vi "TLB Native Dynamic Events ver 0.07.vi"() -> ()   [LabVIEW 2018]
uses:
  Labview Training Phase 2/Enum Controls/States for Action Engine.ctl
  Type def/TLB event states.ctl
  Type def/TLB MHL States.ctl
  <vilib>/Studica/Studica Toolkit/Background/I2C Channel.ctl
  <vilib>/Studica/Studica Toolkit/NavX/NavX.lvlib
  <vilib>/myRIO/Common/Instrument Driver Framework/myRIO v1.0/AI/typedefs/AI Channels Enum.ctl
  <vilib>/myRIO/Common/Instrument Driver Framework/myRIO v1.0/AI/typedefs/AI Channels List.ctl
  Type def/Type def.ctl
  Type def/Motor Control Cluster.ctl
  <vilib>/Studica/Studica Blackhawk/Blackhawk.lvlib
  <vilib>/userdefined/High Color/IMAQdx.ctl
  Underlying VI's/Webcam FGV Low level ver/State control.ctl
  <vilib>/Studica/Studica Toolkit/Background/Mxp Selection.ctl
  <vilib>/ptbypt/NI_PtbyPt.lvlib
  <vilib>/Studica/Studica Toolkit/Background/DIO Channel.ctl
  <vilib>/addons/control/pid/NI_PID_pid.lvlib
  <vilib>/addons/control/pid/pid.llb/PID (DBL).vi
panel:
  in  "STOP":bool
  out "DIO 0":bool
  out "DIO 1":bool
  out "Limit Switch Array":bool[](array[boolean])
  out "Speed and distance cluster":T1
  out "error out":errorcluster
  out "Blackhawk loop":i32
  out "NavX Loop":i32
  out "Sensor Loop":i32
  out "User event loop":i32
  out "Event handling loop":i32
  out "Main Loop":i32
  out "Status loop":i32
  out "L/R average":fxp<+,64,64>
  out "Right Ultrasonic":fxp<+,64,16>
  out "Left Ultrasonic":fxp<+,64,16>
  out "Object detection count":T2
  out "Camera error":errorcluster
  out "Right IR Sensor":dbl
  out "Left IR Sensor":dbl
  in  "Servo Angle":u8(slide) scale=0.0..180.0
  in  "On/Off":bool
  out "Blackhawk error":errorcluster
  out "Image Out":T3(plugin-control)
  out "element":T4
  out "Action Queue Items":i32
  out "State Logic Queue Items":i32
  out "Action Queues items":string[](array[string])=["Hardware reset", "Software reset", ""]
  out "State logic":T5=enum."Task 2"
  out "Action State":string
  in  "Tasks Selector":string(combo)="Wall following"
  out "Yaw":dbl
  out "NavX Info Out":T7
  out "LinearAcceleration":T8
  out "Displacement":T9
  out "YRPHfH":T10
  out "Object detected":bool
  in  "NavX Zero Yaw":bool
  # "Camera Status Loop"
  # "TLB FRAMEWORK STATUS"
  # "Test Programme written by Calvin Loke    Dated: 28 Aug 2019\nTest Programme revised by Dr Alex See   Dated 30 Aug 2019\n\nProgramme version:   TLB Native Dynamic Events ver 0.04b.vi"
  # "Sequence of Actions"
  # "Continuous (Repeated)"
  # "Motor Control Loop"
  # "Sensor data"
  # "Blackhawk status"
  # "System Health Status Update"
  # "NAVX Control Loop"
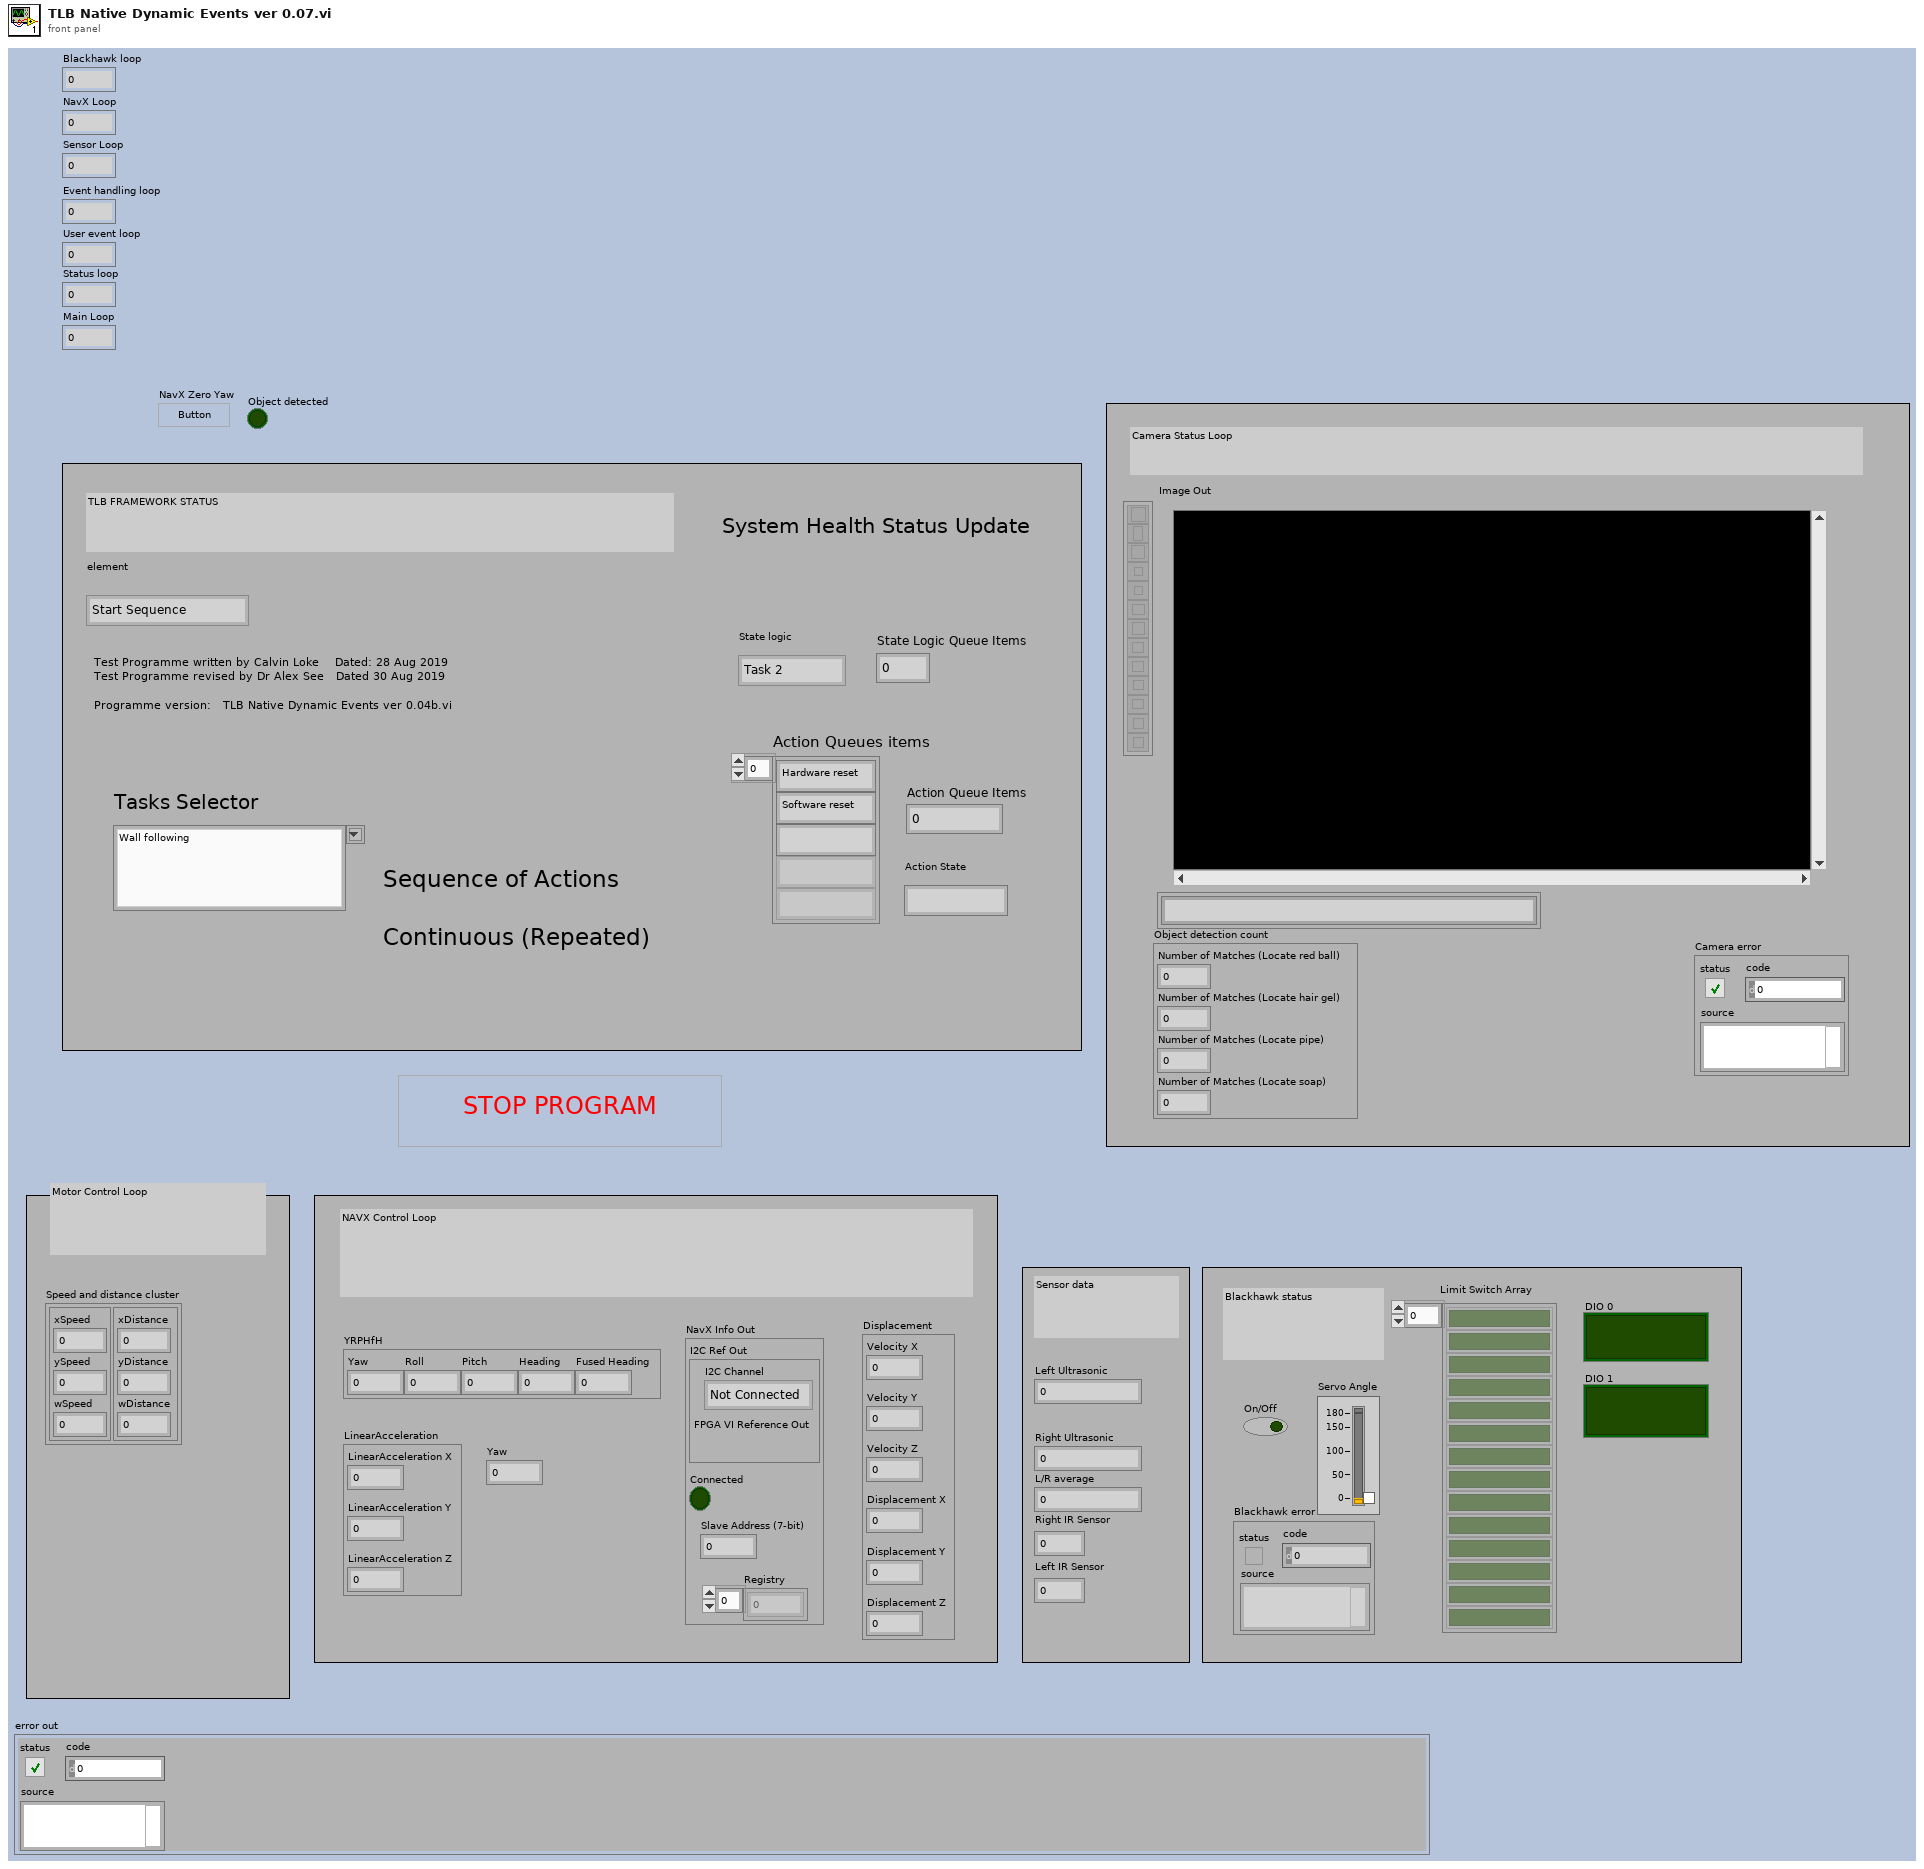
[diagram p1: front panel]
types:
  T1 = cluster{cluster{"xSpeed":dbl, "ySpeed":dbl, "wSpeed":dbl}, cluster{"xDistance":dbl, "yDistance":dbl, "wDistance":dbl}}
  T2 = cluster{"Number of Matches (Locate red ball)":i32, "Number of Matches (Locate hair gel)":i32, "Number of Matches (Locate pipe)":i32, "Number of Matches (Locate soap)":i32}
  T3 = typedef "IMAQ Image.ctl" = refnum<image>
  T4 = typedef "TLB event states.ctl" = enum16{"Start Sequence", "Exit", "Start Task 1", "Start Task 2", "Start Task 3", "Start Task 4", "Camera vision", "Wall follow mode", "Idle", "Start Drive Straight"}
  T5 = typedef "TLB MHL States.ctl" = enum16{"None", "Startup", "Idle", "Processing", "Shutdown", "Reset", "Task 1", "Task 2", "Task 3", "Task 4", "Task 4a", "Task 4b", "Task 4c", "Task 4d", "Task 4e", "Task 4f", "Task 4g", "Task 4h", "Acquire image", "Wall follow mode", "Autodrive", "Autodrive a"}
  T6 = typedef "I2C Channel.ctl" = enum16{"Not Connected", "A", "B"}
  T7 = cluster{"I2C Ref Out":cluster{"I2C Channel":T6, "FPGA VI Reference Out":refnum<k20>}, "Connected":bool, "Slave Address (7-bit)":u8, "Registry":u8[]}
  T8 = cluster{"LinearAcceleration X":dbl, "LinearAcceleration Y":dbl, "LinearAcceleration Z":dbl}
  T9 = cluster{"Velocity X":dbl, "Velocity Y":dbl, "Velocity Z":dbl, "Displacement X":dbl, "Displacement Y":dbl, "Displacement Z":dbl}
  T10 = cluster{"Yaw":dbl, "Roll":dbl, "Pitch":dbl, "Heading":dbl, "Fused Heading":dbl}
  T11 = typedef "States for Action Engine.ctl" = enum16{"Initialize", "Write", "Read"}
  T12 = typedef "DIO Channel.ctl" = enum16{"Not Connected", "A/DIO1", "A/DIO2", "A/DIO3", "A/DIO4", "A/DIO5", "A/DIO6", "A/DIO7", "A/DIO13", "B/DIO1", "B/DIO2", "B/DIO3", "B/DIO4", "B/DIO5", "B/DIO6", "B/DIO7", "B/DIO13", "C/DIO0", "C/DIO1", "C/DIO2", "C/DIO3", "C/DIO4", "C/DIO5", "C/DIO6", "C/DIO7"}
  T13 = typedef "Motor Control Cluster.ctl" = cluster{"Vx":dbl, "Vy":dbl, "Vw":dbl}
  T14 = typedef "Type def.ctl" = cluster{"Front Ultrasonic Obstruct":bool, "Left Ultrasonic Obstruct":bool, "Right Ultrasonic Obstruct ":bool}
  T15 = typedef "Mxp Selection.ctl" = enum16{"MXP A", "MXP B"}
  T16 = cluster{"proportional gain (Kc)":dbl, "integral time (Ti, min)":dbl, "derivative time (Td, min)":dbl}
  T17 = typedef "State control.ctl" = enum16{"Initialise", "Start camera", "Continuous Acquisition ", "Stop camera", "Dispose all"}
  T18 = typedef "IMAQdx.ctl" = refnum<k21>
  T19 = cluster{"xTargetSpeed":dbl, "yTargetSpeed":dbl, "wTargetSpeed":dbl}
  T20 = cluster{"DIO Channel":T12, "FPGA VI Reference Out":refnum<k20>}
  T21 = cluster{"xDistance":dbl, "yDistance":dbl, "wDistance":dbl}
  T22 = typedef "AI Channels List.ctl" = T23[]
  T23 = typedef "AI Channels Enum.ctl" = enum16{"Not Connected", "AudioIn/Left", "AudioIn/Right", "C/AI0", "C/AI1", "A/AI0", "A/AI1", "A/AI2", "A/AI3", "A/AI4", "A/AI5", "A/AI6", "A/AI7", "B/AI0", "B/AI1", "B/AI2", "B/AI3", "B/AI4", "B/AI5", "B/AI6", "B/AI7", "AI/AI0", "AI/AI1", "AI/AI2", "AI/AI3", "A/AI0 (DIFF)", "A/AI1 (DIFF)", "A/AI2 (DIFF)", "A/AI3 (DIFF)", "B/AI0 (DIFF)", "B/AI1 (DIFF)", "B/AI2 (DIFF)", "B/AI3 (DIFF)"}
  T24 = cluster{"I2C Channel":T6, "FPGA VI Reference Out":refnum<k20>}
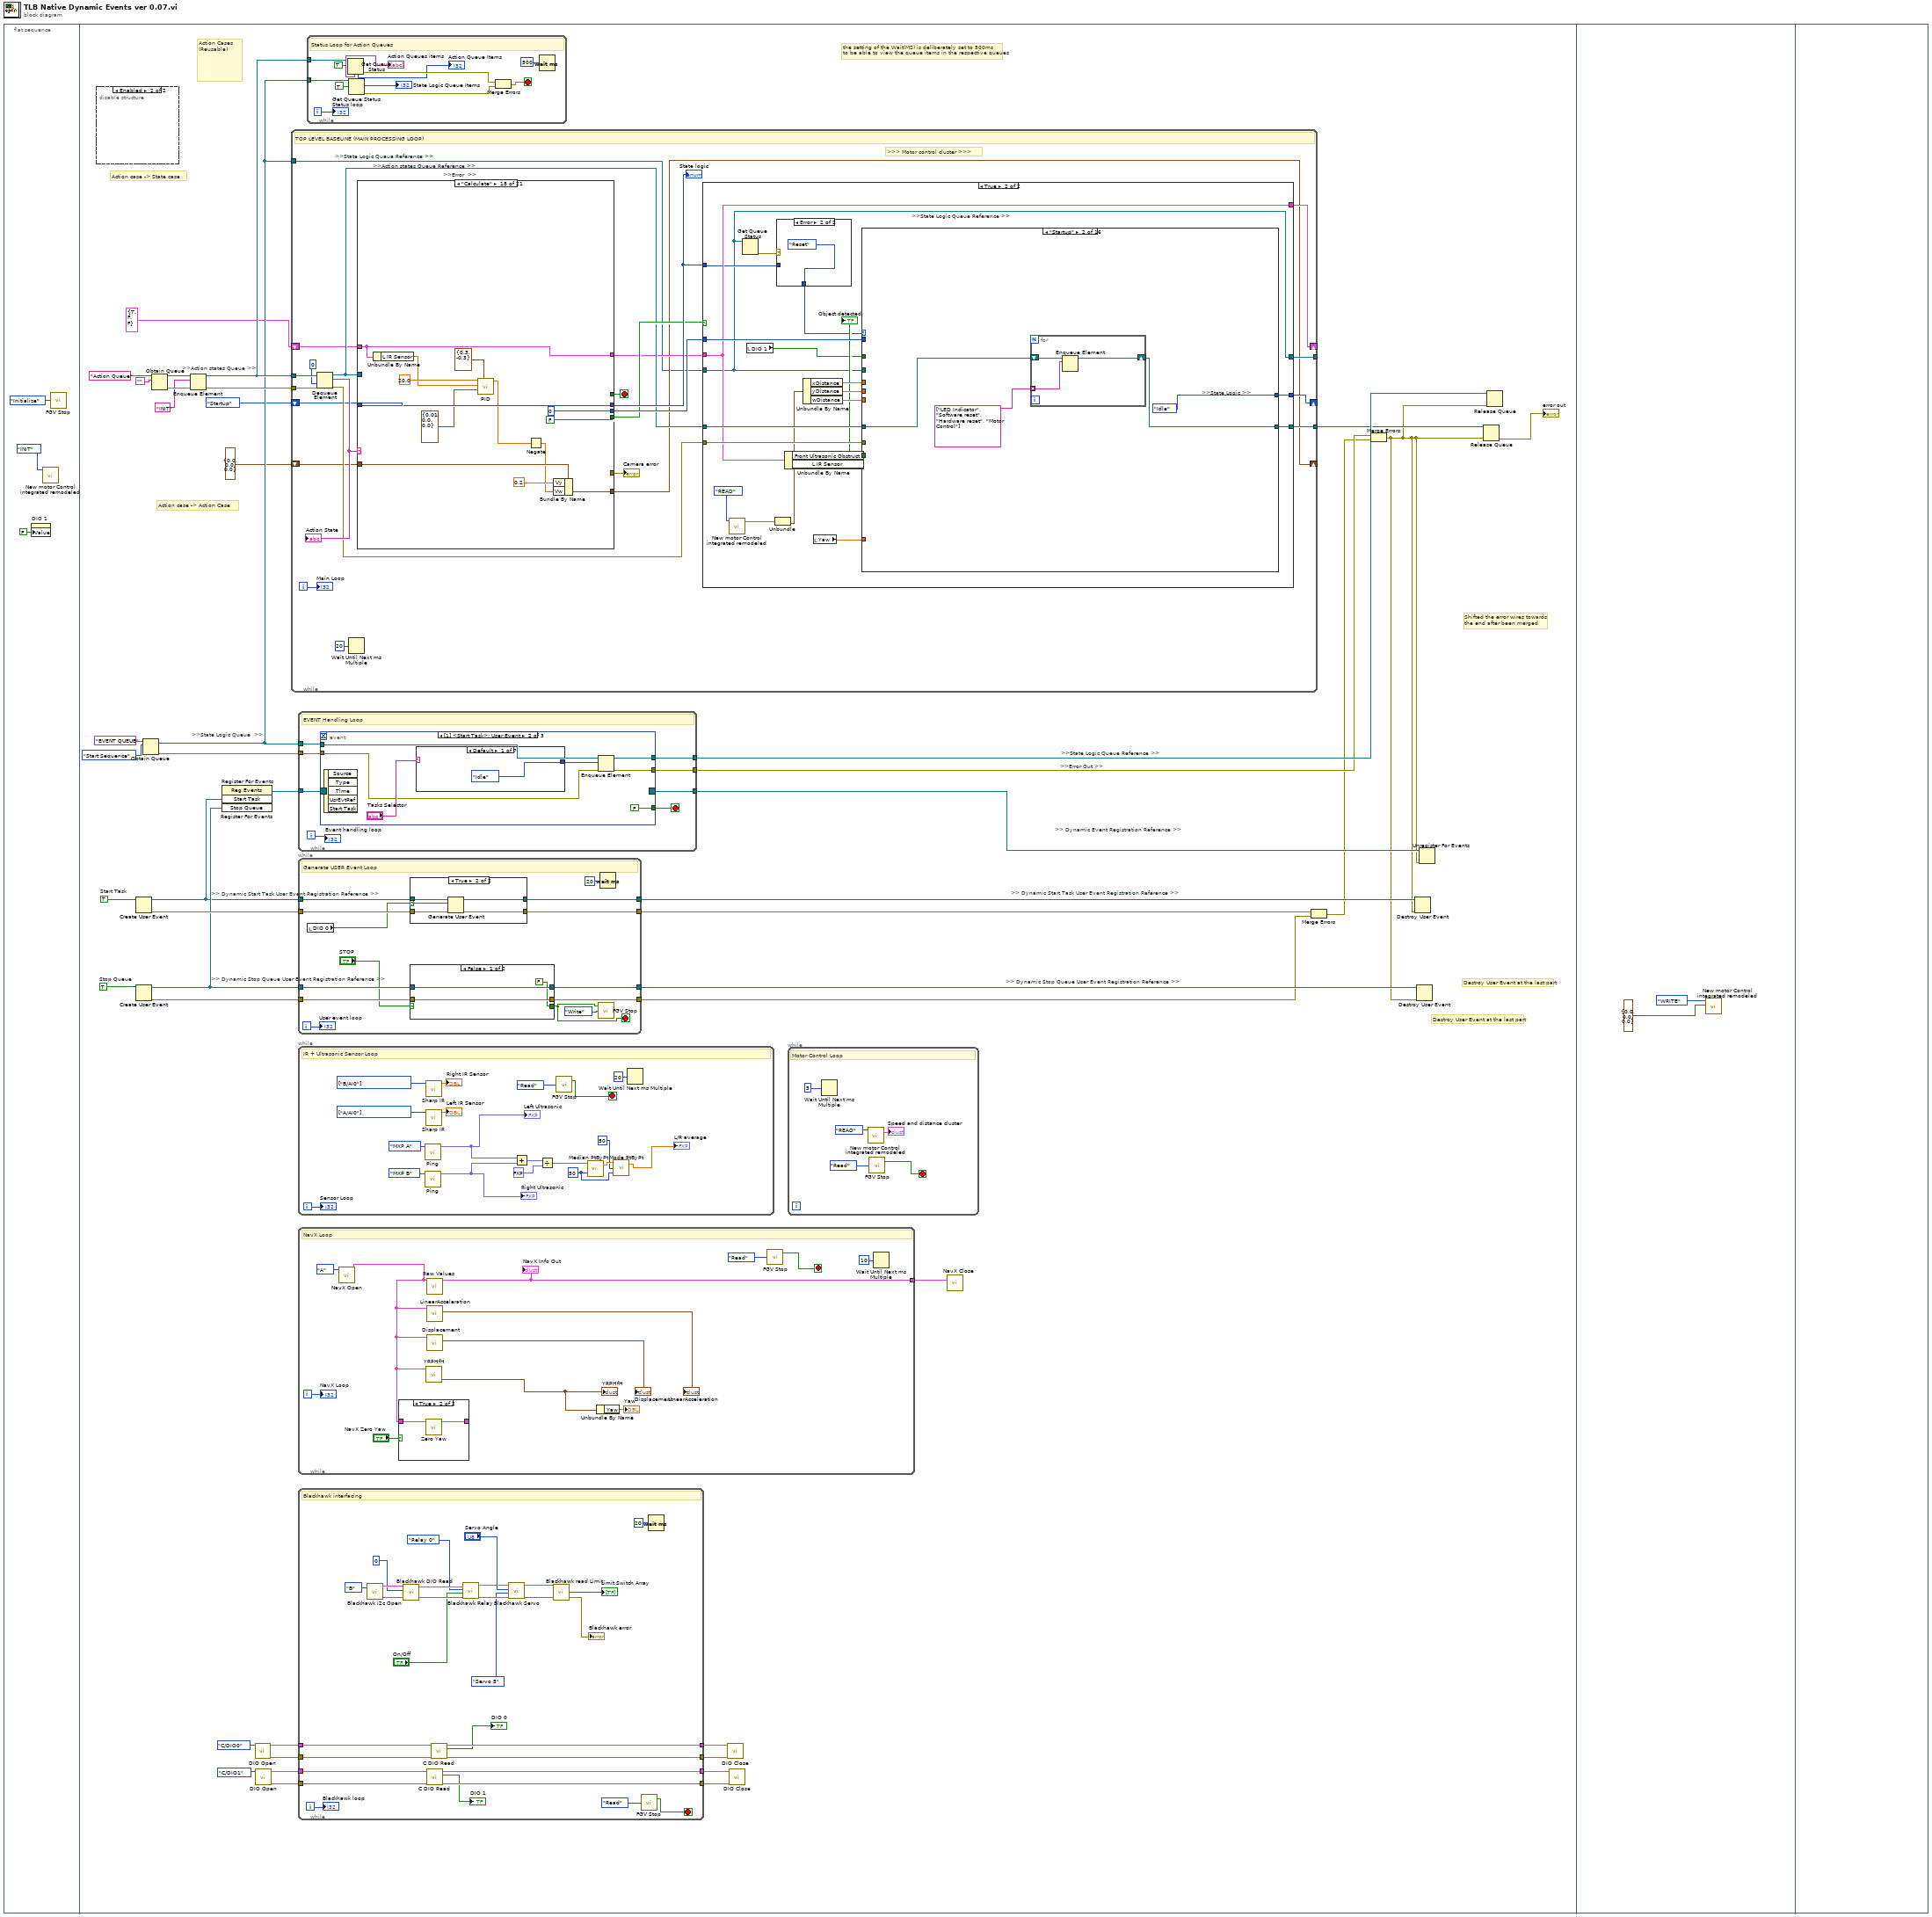
[diagram p0: block diagram]
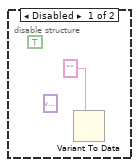
[diagram p3: hidden frame]
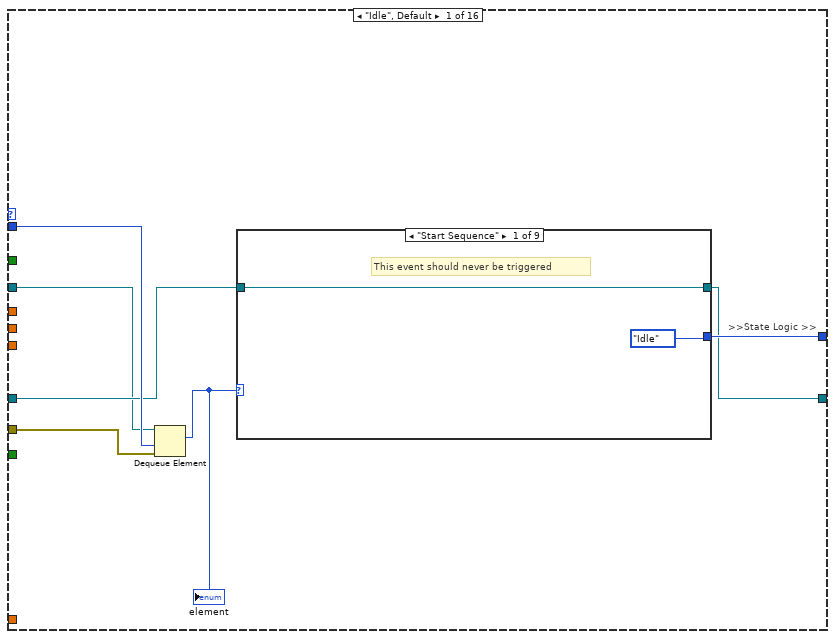
[diagram p6: hidden frame]
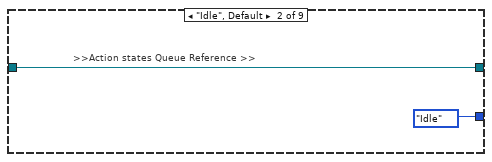
[diagram p7: hidden frame]
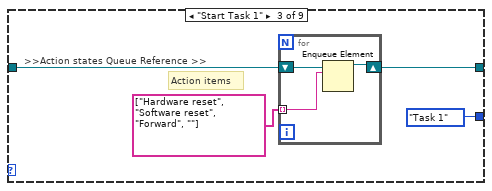
[diagram p8: hidden frame]
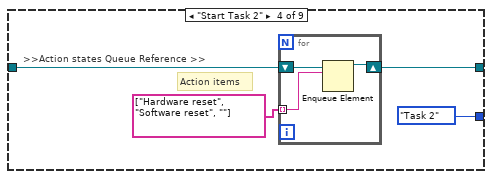
[diagram p9: hidden frame]
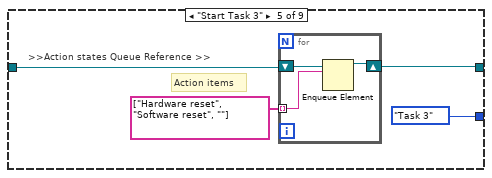
[diagram p10: hidden frame]
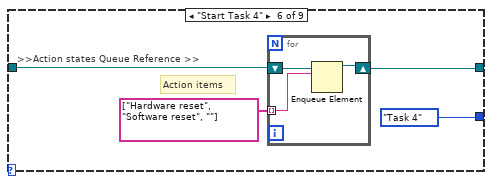
[diagram p11: hidden frame]
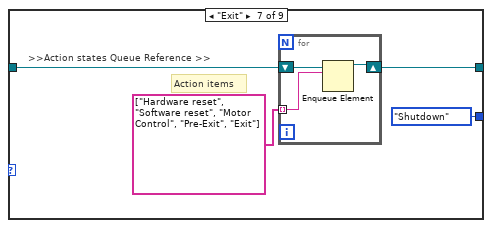
[diagram p12: hidden frame]
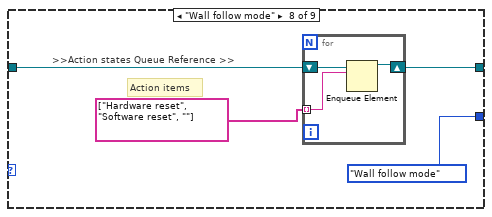
[diagram p13: hidden frame]
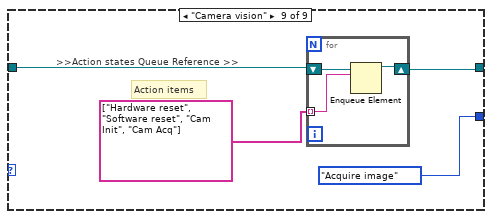
[diagram p14: hidden frame]
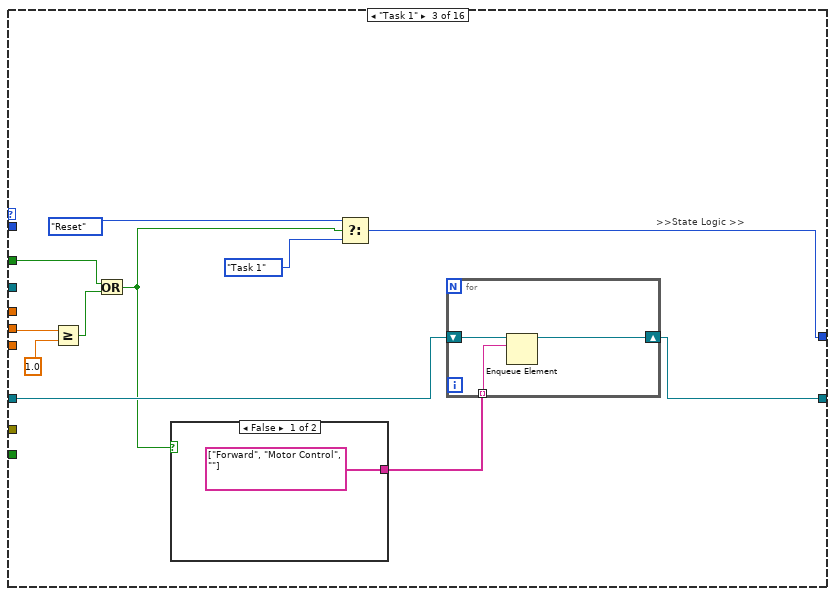
[diagram p15: hidden frame]
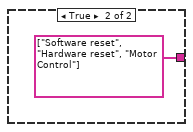
[diagram p16: hidden frame]
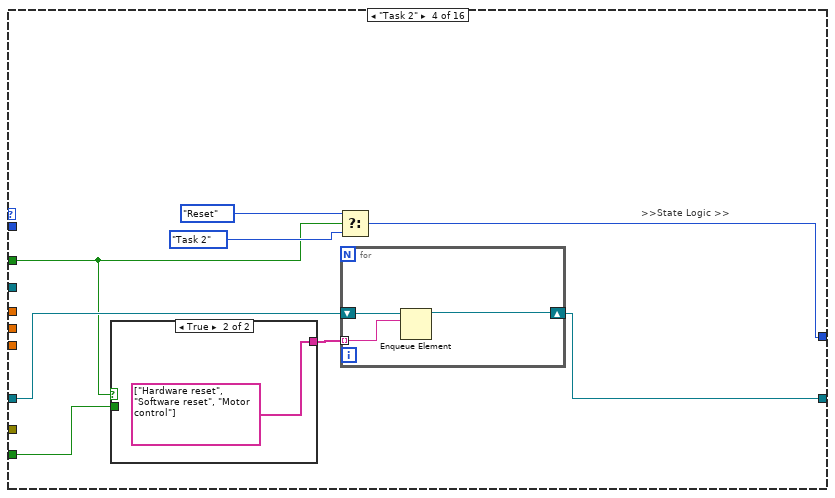
[diagram p17: hidden frame]
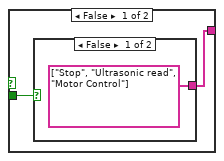
[diagram p18: hidden frame]
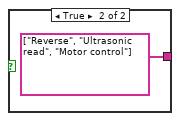
[diagram p19: hidden frame]
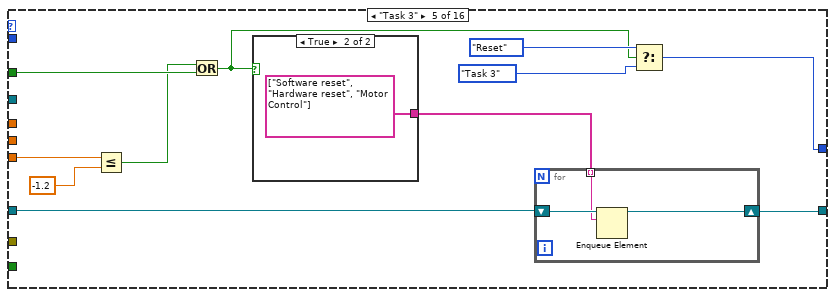
[diagram p20: hidden frame]
diagram:
  n1 = flat-sequence {
    frame #0 {
      n2 = property on="DIO 1" class="Bool (strict)"("Value"=FALSE ("DIO 1")) -> ()  [unwired: 2 in, 2 out]
      n3 = call "New motor Control integrated remodeled.vi"("States"=enum16{"RESET ENCODER", "WRITE", "READ", "INIT"}."INIT") -> ()  [unwired: 4 in, 2 out]
      n4 = call "FGV Stop.vi"("Init/Read/Write State"=States_for_Action_Engine."Initialize") -> ()  [unwired: 2 in, 2 out]
    }
    frame #1 {
      w46 = TRUE  # Stop Queue
      w45 = TRUE  # Start Task
      # "Action case -> Action Case"
      # "Action case -> State case"
      # "the setting of the Wait(MS) is deliberately set to 500ms\nto be able to view the queue items in the respective queues"
      # "Action Cases\n(Reusable)"
      # ">>Error Out >>"
      # ">> Dynamic Stop Queue User Event Registration Reference >>"
      # ">> Dynamic Start Task User Event Registration Reference >>"
      # ">> Dynamic Stop Queue User Event Registration Reference >>"
      # ">> Dynamic Start Task User Event Registration Reference >>"
      # ">> Dynamic Event Registration Reference >>"
      # ">>Action states Queue >>"
      # ">>State Logic Queue  >>"
      # ">>State Logic Queue Reference >>"
      # "Destroy User Event at the last part"
      # "Destroy User Event at the last part"
      # "Shifted the error wires towards\nthe end after been merged"
      n5 = disable-structure shown="Enabled" {
        frame Disabled {
          (unwired) variant
          (unwired) TRUE
          n6 = Variant To Data(type="") -> ()  [unwired: 2 in, 2 out]
        }
        frame Enabled {
        }
      }
      n7 = Create User Event(user event datatype=w45) -> (user event=w37:refnum<user-event>, error out=w42:errorcluster)  [unwired: 1 in]
      n8 = Create User Event(user event datatype=w46) -> (user event=w38:refnum<user-event>, error out=w41:errorcluster)  [unwired: 1 in]
      n9 = Obtain Queue(name (unnamed)="EVENT QUEUE", element data type=TLB_event_states."Start Sequence" ("Enum")) -> (queue out=w22:refnum<queue>, error out=w28:errorcluster)  [unwired: 3 in, 1 out]
      n10 = Obtain Queue(name (unnamed)="Action Queue", element data type="") -> (queue out=w31:refnum<queue>, error out=w27:errorcluster)  [unwired: 3 in, 1 out]
      n11 = Enqueue Element(queue=w31, element="INIT", error in (no error)=w27) -> (queue out=w23:refnum<queue>, error out=w26:errorcluster)  [unwired: 1 in, 1 out]
      n12 = register-events "Register For Events"(w37, w38) -> (reference out=w36:refnum<event-registration>)  [unwired: 2 in, 1 out]
      n13 = call <vilib>:"DIO Open.vi"("DIO Channel"=DIO_Channel."C/DIO0") -> ("error out"=w10:errorcluster, "DIO Info Out"=w16:T20)  [unwired: 9 in]
      n14 = call <vilib>:"DIO Open.vi"("DIO Channel"=DIO_Channel."C/DIO1") -> ("error out"=w8:errorcluster, "DIO Info Out"=w12:T20)  [unwired: 9 in]
      n15 = while {
        tunnel: w22 -> [w131]
        shift-right: [w145] -> _
        shift-left: TLB_MHL_States."Startup" ("Enum") -> [w139]
        tunnel: w23 -> [w150]
        tunnel: w26 -> [w148]
        tunnel: [w147] -> _
        tunnel: [w146] -> w6
        shift-right: [w136] -> _
        shift-left: T14 {"Front Ultrasonic Obstruct"=TRUE, "Left Ultrasonic Obstruct"=FALSE, "Right Ultrasonic Obstruct "=FALSE} -> [w138]
        shift-right: [w134] -> _
        shift-left: T13 {"Vx"=0.0, "Vy"=0.0, "Vw"=0.0} -> [w135]
        i -> [w132]
        stop <- w129 stop-if-true
        # ">>> Motor control cluster >>>"
        # ">>Error  >>"
        # ">>Action states Queue Reference >>"
        # ">>State Logic Queue Reference >>"
        # "TOP LEVEL BASELINE (MAIN PROCESSING LOOP)"
        n16 = Dequeue Element(queue=w150, timeout in ms (-1)=0, error in (no error)=w148) -> (queue out=w140:refnum<queue>, element=w149:string, error out=w141:errorcluster)  [unwired: 1 out]
        "Action State" <- w149
        n17 = Wait Until Next ms Multiple(millisecond multiple=u32 20) -> ()  [unwired: 1 out]
        n18 = case shown="\"Calculate\"" w149 {
          tunnel: [w402 w414 w419 w426 w434 w443 w451 w457 w467 w474 w480 w490 w500 TLB_MHL_States."Shutdown" ("Enum") w511 w521 w525 w540 w552 w561 w575] -> w151
          tunnel: [w406 0 0 0 0 0 0 0 0 0 0 0 0 0 0 0 0 0 0 0 0] -> w144
          tunnel: [TRUE FALSE FALSE FALSE FALSE FALSE FALSE FALSE FALSE FALSE FALSE FALSE FALSE FALSE FALSE FALSE FALSE FALSE FALSE FALSE FALSE] -> w143
          tunnel: w140 -> [_ _ _ _ _ _ _ _ _ _ _ _ _ _ _ _ _ _ _ _ _]
          tunnel: w139 -> [w402 w414 w419 w426 w434 w443 w451 w457 w467 w474 w480 w490 w500 _ w511 w521 w525 w540 w552 w561 w575]
          tunnel: w138 -> [w404 w411 w416 w423 w431 w439 w447 w455 w463 w471 w481 w487 w496 w503 w512 w520 w528 w541 w553 w560 w571]
          tunnel: [w404 w411 w416 w423 w431 w439 w447 w455 w463 w471 w481 w486 w496 w503 w512 w517 w527 w541 w553 w560 w571] -> w137
          tunnel: w135 -> [w403 w410 w415 w421 w429 w437 w446 w453 w462 w469 w477 w484 w495 w502 w508 w514 w522 w536 w551 w564 w572]
          tunnel: [w403 w410 w415 w422 w430 w438 w445 w454 w461 w470 w477 w484 w493 w502 w508 w514 w522 w537 w551 w564 w572] -> w134
          tunnel: [_ _ _ _ _ _ _ _ _ _ _ _ _ _ _ _ _ _ w542 w556 w565] -> w133
          tunnel: [_ _ _ _ _ _ _ _ _ _ _ _ _ TRUE _ _ _ _ _ _ _] -> w129
          frame "No action", Default {
            n19 = case shown="\"Startup\", Default" w402 {
              tunnel: [0 100] -> w406
              frame "Startup", Default {
              }
              frame "Idle" {
              }
            }
          }
          frame "Init" {
            # ">>State Logic  >>"
            n20 = local write "Servo Angle"(u8 90 ("Servo Angle")) -> ()
          }
          frame "LED Indicator" {
          }
          frame "Forward" {
            n21 = local write "NavX Zero Yaw"(FALSE ("NavX Zero Yaw")) -> ()
            n22 = Bundle By Name(cluster=w421, "Vy"=0.6) -> (w422:T13)
          }
          frame "Reverse" {
            n23 = local write "NavX Zero Yaw"(FALSE ("NavX Zero Yaw")) -> ()
            n24 = Bundle By Name(cluster=w429, "Vy"=-0.6) -> (w430:T13)
          }
          frame "Right" {
            n25 = local write "NavX Zero Yaw"(FALSE ("NavX Zero Yaw")) -> ()
            n26 = Bundle By Name(cluster=w437, "Vx"=0.6) -> (w438:T13)
          }
          frame "Left" {
            n27 = Bundle By Name(cluster=w446, "Vx"=-0.6) -> (w445:T13)
            n28 = local write "NavX Zero Yaw"(FALSE ("NavX Zero Yaw")) -> ()
          }
          frame "Rotate CW" {
            n29 = local write "NavX Zero Yaw"(FALSE ("NavX Zero Yaw")) -> ()
            n30 = Bundle By Name(cluster=w453, "Vw"=-0.3) -> (w454:T13)
          }
          frame "Rotate ACW" {
            n31 = local write "NavX Zero Yaw"(FALSE ("NavX Zero Yaw")) -> ()
            n32 = Bundle By Name(cluster=w462, "Vw"=0.15) -> (w461:T13)
          }
          frame "Stop" {
            w468 = 0.0
            n33 = local write "NavX Zero Yaw"(FALSE ("NavX Zero Yaw")) -> ()
            n34 = Bundle By Name(cluster=w469, "Vx"=w468, "Vy"=w468, "Vw"=w468) -> (w470:T13)
          }
          frame "Motor control" {
            n35 = call "New motor Control integrated remodeled.vi"("States"=enum16{"RESET ENCODER", "WRITE", "READ", "INIT"}."WRITE", "Target Speed"=w477) -> ()  [unwired: 3 in, 2 out]
          }
          frame "Software reset" {
            w485 = FALSE ("NavX Zero Yaw")
            n36 = Wait (ms)(milliseconds to wait=u32 20) -> ()  [unwired: 1 out]
            n37 = local write "NavX Zero Yaw"(w485) -> ()
            n38 = Bundle By Name(cluster=w487, "Front Ultrasonic Obstruct"=w485, "L IR Sensor"=0.0) -> (w486:T14)
          }
          frame "Hardware reset" {
            w494 = 0.0
            n39 = Wait (ms)(milliseconds to wait=u32 20) -> ()  [unwired: 1 out]
            n40 = local write "NavX Zero Yaw"(TRUE ("NavX Zero Yaw")) -> ()
            n41 = call "New motor Control integrated remodeled.vi"("States"=enum16{"RESET ENCODER", "WRITE", "READ", "INIT"}."RESET ENCODER") -> ()  [unwired: 4 in, 2 out]
            n42 = Bundle By Name(cluster=w495, "Vx"=w494, "Vy"=w494, "Vw"=w494) -> (w493:T13)
          }
          frame "Exit" {
          }
          frame "Pre-Exit" {
            n43 = call "New motor Control integrated remodeled.vi"("States"=enum16{"RESET ENCODER", "WRITE", "READ", "INIT"}."INIT") -> ()  [unwired: 4 in, 2 out]
          }
          frame "Ultrasonic read" {
            # "Object detection"
            n44 = local read "L/R average"() -> (w513:fxp<+,64,64>)
            n45 = Less Or Equal?(x=w513, y=35.0) -> (x <= y?=w515:bool)
            n46 = Bundle By Name(cluster=w520, "Front Ultrasonic Obstruct"=w515) -> (w517:T14)
          }
          frame "IR Sensor Read" {
            n47 = local read "Left IR Sensor"() -> (w526:dbl)
            n48 = Bundle By Name(cluster=w528, "L IR Sensor"=w526) -> (w527:T14)
          }
          frame "Calculate" {
            n49 = Unbundle By Name(w541) -> ("L IR Sensor"=w533:dbl)
            n50 = call-poly <vilib>:"PID.vi"("output range"=cluster{"output high":dbl, "output low":dbl} {"output high"=0.3, "output low"=-0.3}, "PID gains"=T16 {"proportional gain (Kc)"=0.01, "integral time (Ti, min)"=0.0, "derivative time (Td, min)"=0.0}, "process variable"=w533, "setpoint"=20.0) -> ("output"=w530:dbl)  [unwired: 6 in, 1 out]
            n51 = Negate(x=w530) -> (-x=w529:dbl)
            n52 = Bundle By Name(cluster=w536, "Vy"=0.2, "Vw"=w529) -> (w537:T13)
          }
          frame "Cam Init" {
            n53 = call "Low-Level Grab.vi"("States"=State_control."Initialise", "Session In"=T18 "cam1") -> ("error out"=w543:errorcluster, "Session Out"=w544:T18)  [unwired: 7 in, 1 out]
            n54 = call "Low-Level Grab.vi"("error in (no error)"=w543, "States"=State_control."Start camera", "Session In"=w544) -> ("error out"=w542:errorcluster)  [unwired: 6 in, 2 out]
            n55 = local write "Servo Angle"(u8 170 ("Servo Angle")) -> ()
          }
          frame "Cam Acq" {
            n56 = call "Low-Level Grab.vi"("States"=State_control."Continuous Acquisition ") -> ("error out"=w557:errorcluster, "Image Out"=w558:T3)  [unwired: 8 in, 1 out]
            n57 = call "All object detection ver2.vi"("Image In"=w558, "error in"=w557) -> ("Image Out"=→"Image Out":T3, "Object detection count"=→"Object detection count":T2, "error out"=w556:errorcluster)
          }
          frame "Cam Exit" {
            n58 = call "Low-Level Grab.vi"("States"=State_control."Stop camera") -> ("error out"=w566:errorcluster, "Session Out"=w568:T18)  [unwired: 8 in, 1 out]
            n59 = local write "Servo Angle"(u8 90 ("Servo Angle")) -> ()
            n60 = call "Low-Level Grab.vi"("error in (no error)"=w566, "States"=State_control."Dispose all", "Session In"=w568) -> ("error out"=w565:errorcluster)  [unwired: 6 in, 2 out]
          }
        }
        "State logic" <- w151
        "Camera error" <- w133
        n61 = case shown="True" w143 {
          tunnel: w151 -> [w154 w159]
          tunnel: w131 -> [w155 w158]
          tunnel: w140 -> [w153 w174]
          tunnel: [w155 w158] -> w147
          tunnel: [w153 w173] -> w146
          tunnel: [w154 w172] -> w145
          tunnel: w141 -> [_ w171]
          tunnel: w144 -> [_ w170]
          tunnel: w137 -> [w152 w164]
          tunnel: [w152 w164] -> w136
          frame False {
          }
          frame True {
            # ">>State Logic Queue Reference >>"
            n62 = call "New motor Control integrated remodeled.vi"("States"=enum16{"RESET ENCODER", "WRITE", "READ", "INIT"}."READ") -> ("Speed and distance cluster"=w163:T1)  [unwired: 4 in, 1 out]
            n63 = Get Queue Status(queue=w158) -> (error out=w157:errorcluster)  [unwired: 2 in, 7 out]
            n64 = local read "DIO 1"() -> (w156:bool)
            n65 = Unbundle(w163) -> (w162:T21)  [unwired: 1 out]
            n66 = case shown="Error" w157 {
              tunnel: [w175 TLB_MHL_States."Reset" ("Enum")] -> w160
              tunnel: w159 -> [w175 _]
              frame No Error {
              }
              frame Error {
              }
            }
            n67 = Unbundle By Name(w164) -> ("Front Ultrasonic Obstruct"=w165:bool)  [unwired: 1 out]
            "Object detected" <- w165
            n68 = Unbundle By Name(w162) -> ("xDistance"=w167:dbl, "yDistance"=w169:dbl, "wDistance"=w168:dbl)
            n69 = local read "Yaw"() -> (w166:dbl)
            n70 = case shown="\"Startup\"" w160 {
              tunnel: w158 -> [w177 _ _ _ _ _ _ _ _ _ _ _ _ _ _ _]
              tunnel: w174 -> [w179 w238 w250 w263 w285 w294 w308 w323 w336 w351 w361 w369 w382 w391 w394 w400]
              tunnel: [w178 w237 w249 w264 w284 w295 w307 w322 w335 w350 w360 w370 w381 w391 w393 w400] -> w173
              tunnel: [w182 TLB_MHL_States."Idle" ("Enum") w252 w265 w281 w298 w310 w321 w337 w349 TLB_MHL_States."Shutdown" ("Enum") w372 w380 TLB_MHL_States."Reset" ("Enum") TLB_MHL_States."Shutdown" ("Enum") TLB_MHL_States."Reset" ("Enum")] -> w172
              tunnel: w171 -> [w180 _ _ _ _ _ _ _ _ _ _ _ _ _ _ _]
              tunnel: w170 -> [w181 _ _ _ _ _ _ _ _ _ _ _ _ _ _ _]
              tunnel: w156 -> [_ _ w247 w262 w279 _ _ _ _ w348 _ w367 w379 _ _ _]
              tunnel: w169 -> [_ _ w244 _ _ _ _ w318 _ _ _ _ _ _ _ _]
              tunnel: w168 -> [_ _ _ _ w276 _ _ _ _ _ _ _ _ _ _ _]
              tunnel: w167 -> [_ _ _ _ _ _ w304 _ w332 _ _ _ _ _ _ _]
              tunnel: w166 -> [_ _ _ _ _ _ _ _ _ _ _ _ _ _ _ _]
              tunnel: w165 -> [_ _ _ w260 _ w292 _ _ _ w347 _ _ _ _ _ _]
              frame "Idle", Default {
                # ">>State Logic >>"
                n71 = Dequeue Element(queue=w177, timeout in ms (-1)=w181, error in (no error)=w180) -> (element=w183:T4)  [unwired: 3 out]
                "element" <- w183
                n72 = case shown="\"Start Sequence\"" w183 {
                  tunnel: [TLB_MHL_States."Idle" ("Enum") TLB_MHL_States."Idle" ("Enum") TLB_MHL_States."Task 1" ("Enum") TLB_MHL_States."Task 2" ("Enum") TLB_MHL_States."Task 3" ("Enum") TLB_MHL_States."Task 4" ("Enum") TLB_MHL_States."Shutdown" ("Enum") TLB_MHL_States."Wall follow mode" ("Enum") TLB_MHL_States."Acquire image" ("Enum")] -> w182
                  tunnel: [w185 w186 w190 w195 w204 w210 w216 w223 w231] -> w178
                  tunnel: w179 -> [w185 w186 w188 w196 w205 w211 w217 w224 w232]
                  frame "Start Sequence" {
                    # "This event should never be triggered"
                  }
                  frame "Idle", Default {
                    # ">>Action states Queue Reference >>"
                  }
                  frame "Start Task 1" {
                    # ">>Action states Queue Reference >>"
                    # "Action items"
                    n73 = for {
                      shift-right: [w194] -> w190
                      shift-left: w188 -> [w193]
                      tunnel: string[] ["Hardware reset", "Software reset", "Forward", ""] -> [w192] mode=indexing
                      n74 = Enqueue Element(queue=w193, element=w192) -> (queue out=w194:refnum<queue>)  [unwired: 2 in, 2 out]
                    }
                  }
                  frame "Start Task 2" {
                    # ">>Action states Queue Reference >>"
                    # "Action items"
                    n75 = for {
                      shift-right: [w201] -> w195
                      shift-left: w196 -> [w200]
                      tunnel: string[] ["Hardware reset", "Software reset", ""] -> [w199] mode=indexing
                      n76 = Enqueue Element(queue=w200, element=w199) -> (queue out=w201:refnum<queue>)  [unwired: 2 in, 2 out]
                    }
                  }
                  frame "Start Task 3" {
                    # ">>Action states Queue Reference >>"
                    # "Action items"
                    n77 = for {
                      shift-right: [w208] -> w204
                      shift-left: w205 -> [w207]
                      tunnel: string[] ["Hardware reset", "Software reset", ""] -> [w206] mode=indexing
                      n78 = Enqueue Element(queue=w207, element=w206) -> (queue out=w208:refnum<queue>)  [unwired: 2 in, 2 out]
                    }
                  }
                  frame "Start Task 4" {
                    # ">>Action states Queue Reference >>"
                    # "Action items"
                    n79 = for {
                      shift-right: [w215] -> w210
                      shift-left: w211 -> [w214]
                      tunnel: string[] ["Hardware reset", "Software reset", ""] -> [w213] mode=indexing
                      n80 = Enqueue Element(queue=w214, element=w213) -> (queue out=w215:refnum<queue>)  [unwired: 2 in, 2 out]
                    }
                  }
                  frame "Exit" {
                    # ">>Action states Queue Reference >>"
                    # "Action items"
                    n81 = for {
                      shift-right: [w222] -> w216
                      shift-left: w217 -> [w221]
                      tunnel: string[] ["Hardware reset", "Software reset", "Motor Control", "Pre-Exit", "Exit"] -> [w220] mode=indexing
                      n82 = Enqueue Element(queue=w221, element=w220) -> (queue out=w222:refnum<queue>)  [unwired: 2 in, 2 out]
                    }
                  }
                  frame "Wall follow mode" {
                    # ">>Action states Queue Reference >>"
                    # "Action items"
                    n83 = for {
                      shift-right: [w229] -> w223
                      shift-left: w224 -> [w228]
                      tunnel: string[] ["Hardware reset", "Software reset", ""] -> [w227] mode=indexing
                      n84 = Enqueue Element(queue=w228, element=w227) -> (queue out=w229:refnum<queue>)  [unwired: 2 in, 2 out]
                    }
                  }
                  frame "Camera vision" {
                    # ">>Action states Queue Reference >>"
                    # "Action items"
                    n85 = for {
                      shift-right: [w236] -> w231
                      shift-left: w232 -> [w235]
                      tunnel: string[] ["Hardware reset", "Software reset", "Cam Init", "Cam Acq"] -> [w234] mode=indexing
                      n86 = Enqueue Element(queue=w235, element=w234) -> (queue out=w236:refnum<queue>)  [unwired: 2 in, 2 out]
                    }
                  }
                }
              }
              frame "Startup" {
                # ">>State Logic >>"
                n87 = for {
                  shift-right: [w242] -> w237
                  shift-left: w238 -> [w243]
                  tunnel: string[] ["LED Indicator", "Software reset", "Hardware reset", "Motor Control"] -> [w241] mode=indexing
                  n88 = Enqueue Element(queue=w243, element=w241) -> (queue out=w242:refnum<queue>)  [unwired: 2 in, 2 out]
                }
              }
              frame "Task 1" {
                # ">>State Logic >>"
                n89 = Greater Or Equal?(x=w244, y=1.0) -> (x >= y?=w245:bool)
                n90 = Or(x=w247, y=w245) -> (x .or. y?=w248:bool)
                n91 = case shown="False" w248 {
                  tunnel: [string[] ["Forward", "Motor Control", ""] string[] ["Software reset", "Hardware reset", "Motor Control"]] -> w251
                  frame False {
                  }
                  frame True {
                  }
                }
                n92 = Select(t=TLB_MHL_States."Reset" ("Enum"), s=w248, f=TLB_MHL_States."Task 1" ("Enum")) -> (s? t:f=w252:T5)
                n93 = for {
                  shift-right: [w258] -> w249
                  shift-left: w250 -> [w259]
                  tunnel: w251 -> [w257] mode=indexing
                  n94 = Enqueue Element(queue=w259, element=w257) -> (queue out=w258:refnum<queue>)  [unwired: 2 in, 2 out]
                }
              }
              frame "Task 2" {
                # ">>State Logic >>"
                n95 = case shown="True" w262 {
                  tunnel: [w269 string[] ["Hardware reset", "Software reset", "Motor control"]] -> w261
                  tunnel: w260 -> [w268 _]
                  frame False {
                    n96 = case shown="False" w268 {
                      tunnel: [string[] ["Stop", "Ultrasonic read", "Motor Control"] string[] ["Reverse", "Ultrasonic read", "Motor control"]] -> w269
                      frame False {
                      }
                      frame True {
                      }
                    }
                  }
                  frame True {
                  }
                }
                n97 = Select(t=TLB_MHL_States."Reset" ("Enum"), s=w262, f=TLB_MHL_States."Task 2" ("Enum")) -> (s? t:f=w265:T5)
                n98 = for {
                  shift-right: [w274] -> w264
                  shift-left: w263 -> [w275]
                  tunnel: w261 -> [w273] mode=indexing
                  n99 = Enqueue Element(queue=w275, element=w273) -> (queue out=w274:refnum<queue>)  [unwired: 2 in, 2 out]
                }
              }
              frame "Task 3" {
                n100 = Less Or Equal?(x=w276, y=-1.2) -> (x <= y?=w277:bool)
                n101 = Or(x=w277, y=w279) -> (x .or. y?=w280:bool)
                n102 = case shown="True" w280 {
                  tunnel: [string[] ["Rotate CW", "Motor Control"] string[] ["Software reset", "Hardware reset", "Motor Control"]] -> w286
                  frame False {
                  }
                  frame True {
                  }
                }
                n103 = for {
                  shift-right: [w288] -> w284
                  shift-left: w285 -> [w289]
                  tunnel: w286 -> [w287] mode=indexing
                  n104 = Enqueue Element(queue=w289, element=w287) -> (queue out=w288:refnum<queue>)  [unwired: 2 in, 2 out]
                }
                n105 = Select(t=TLB_MHL_States."Reset" ("Enum"), s=w280, f=TLB_MHL_States."Task 3" ("Enum")) -> (s? t:f=w281:T5)
              }
              frame "Task 4" {
                n106 = case shown="True" w292 {
                  tunnel: [string[] ["Forward", "Ultrasonic read", "Motor Control"] string[] ["Stop", "Hardware reset", "Software reset", "Motor Control"]] -> w293
                  frame False {
                  }
                  frame True {
                  }
                }
                n107 = for {
                  shift-right: [w302] -> w295
                  shift-left: w294 -> [w303]
                  tunnel: w293 -> [w301] mode=indexing
                  n108 = Enqueue Element(queue=w303, element=w301) -> (queue out=w302:refnum<queue>)  [unwired: 2 in, 2 out]
                }
                n109 = Select(t=TLB_MHL_States."Task 4a" ("Enum"), s=w292, f=TLB_MHL_States."Task 4" ("Enum")) -> (s? t:f=w298:T5)
              }
              frame "Task 4a" {
                n110 = Greater Or Equal?(x=w304, y=0.5) -> (x >= y?=w306:bool)
                n111 = case shown="True" w306 {
                  tunnel: [string[] ["Right", "Motor Control"] string[] ["Stop", "Hardware reset", "Software reset", "Motor Control"]] -> w309
                  frame False {
                  }
                  frame True {
                  }
                }
                n112 = for {
                  shift-right: [w316] -> w307
                  shift-left: w308 -> [w317]
                  tunnel: w309 -> [w315] mode=indexing
                  n113 = Enqueue Element(queue=w317, element=w315) -> (queue out=w316:refnum<queue>)  [unwired: 2 in, 2 out]
                }
                n114 = Select(t=TLB_MHL_States."Task 4b" ("Enum"), s=w306, f=TLB_MHL_States."Task 4a" ("Enum")) -> (s? t:f=w310:T5)
              }
              frame "Task 4b" {
                n115 = Greater Or Equal?(x=w318, y=0.75) -> (x >= y?=w319:bool)
                n116 = case shown="False" w319 {
                  tunnel: [string[] ["Forward", "Motor control"] string[] ["Stop", "Hardware reset", "Software reset"]] -> w324
                  frame False {
                  }
                  frame True {
                  }
                }
                n117 = for {
                  shift-right: [w330] -> w322
                  shift-left: w323 -> [w331]
                  tunnel: w324 -> [w329] mode=indexing
                  n118 = Enqueue Element(queue=w331, element=w329) -> (queue out=w330:refnum<queue>)  [unwired: 2 in, 2 out]
                }
                n119 = Select(t=TLB_MHL_States."Task 4c" ("Enum"), s=w319, f=TLB_MHL_States."Task 4b" ("Enum")) -> (s? t:f=w321:T5)
              }
              frame "Task 4c" {
                n120 = Less Or Equal?(x=w332, y=-0.65) -> (x <= y?=w333:bool)
                n121 = case shown="False" w333 {
                  tunnel: [string[] ["Left", "Motor Control"] string[] ["Stop", "Hardware reset", "Software reset", "Motor Control"]] -> w338
                  frame False {
                  }
                  frame True {
                  }
                }
                n122 = for {
                  shift-right: [w344] -> w335
                  shift-left: w336 -> [w345]
                  tunnel: w338 -> [w343] mode=indexing
                  n123 = Enqueue Element(queue=w345, element=w343) -> (queue out=w344:refnum<queue>)  [unwired: 2 in, 2 out]
                }
                n124 = Select(t=TLB_MHL_States."Task 4d" ("Enum"), s=w333, f=TLB_MHL_States."Task 4c" ("Enum")) -> (s? t:f=w337:T5)
              }
              frame "Task 4d" {
                n125 = Or(x=w348, y=w347) -> (x .or. y?=w346:bool)
                n126 = case shown="True" w346 {
                  tunnel: [string[] ["Forward", "Ultrasonic Read", "Motor Control"] string[] ["Stop", "Hardware reset", "Software reset", "Motor Control"]] -> w352
                  frame False {
                  }
                  frame True {
                  }
                }
                n127 = for {
                  shift-right: [w358] -> w350
                  shift-left: w351 -> [w359]
                  tunnel: w352 -> [w357] mode=indexing
                  n128 = Enqueue Element(queue=w359, element=w357) -> (queue out=w358:refnum<queue>)  [unwired: 2 in, 2 out]
                }
                n129 = Select(t=TLB_MHL_States."Startup" ("Enum"), s=w346, f=TLB_MHL_States."Task 4d" ("Enum")) -> (s? t:f=w349:T5)
              }
              frame "Reset" {
                n130 = for {
                  shift-right: [w365] -> w360
                  shift-left: w361 -> [w366]
                  tunnel: string[] ["Software reset", "Hardware reset", "Motor Control"] -> [w364] mode=indexing
                  n131 = Enqueue Element(queue=w366, element=w364) -> (queue out=w365:refnum<queue>)  [unwired: 2 in, 2 out]
                }
              }
              frame "Wall follow mode" {
                n132 = case shown="False" w367 {
                  tunnel: [string[] ["IR Sensor Read", "Calculate", "Forward", "Motor Control"] string[] ["Hardware reset", "Software reset", "Motor Control"]] -> w368
                  frame False {
                  }
                  frame True {
                  }
                }
                n133 = for {
                  shift-right: [w377] -> w370
                  shift-left: w369 -> [w378]
                  tunnel: w368 -> [w376] mode=indexing
                  n134 = Enqueue Element(queue=w378, element=w376) -> (queue out=w377:refnum<queue>)  [unwired: 2 in, 2 out]
                }
                n135 = Select(t=TLB_MHL_States."Idle" ("Enum"), s=w367, f=TLB_MHL_States."Wall follow mode" ("Enum")) -> (s? t:f=w372:T5)
              }
              frame "Acquire image" {
                n136 = case shown="True" w379 {
                  tunnel: [string[] ["Cam Acq"] string[] ["Hardware reset", "Software reset", "Cam Exit", ""]] -> w383
                  frame False {
                  }
                  frame True {
                  }
                }
                n137 = for {
                  shift-right: [w389] -> w381
                  shift-left: w382 -> [w390]
                  tunnel: w383 -> [w388] mode=indexing
                  n138 = Enqueue Element(queue=w390, element=w388) -> (queue out=w389:refnum<queue>)  [unwired: 2 in, 2 out]
                }
                n139 = Select(t=TLB_MHL_States."Idle" ("Enum"), s=w379, f=TLB_MHL_States."Acquire image" ("Enum")) -> (s? t:f=w380:T5)
              }
              frame "Processing" {
              }
              frame "Shutdown" {
                # ">>State Logic >>"
                n140 = for {
                  shift-right: [w398] -> w393
                  shift-left: w394 -> [w399]
                  tunnel: string[] ["Software reset", "Hardware reset", "Motor Control", "Cam Exit", "Pre-Exit", "Exit"] -> [w397] mode=indexing
                  n141 = Enqueue Element(queue=w399, element=w397) -> (queue out=w398:refnum<queue>)  [unwired: 2 in, 2 out]
                }
              }
              frame "None" {
              }
            }
          }
        }
        "Main Loop" <- w132
      }
      n142 = while {
        tunnel: w36 -> [w583]
        tunnel: [w582] -> w35
        tunnel: w22 -> [w580]
        tunnel: [w579] -> w34
        tunnel: w28 -> [w578]
        tunnel: [w577] -> w25
        i -> [w576]
        stop <- w581 stop-if-true
        # "EVENT Handling Loop"
        n143 = event shown="[1] <Start Task>: User Event" {
          selector: w583 -> [_ _ _]
          dyn-events: [_ _ _] -> w582
          timeout: _ -> [_ _ _]
          tunnel: [FALSE FALSE w609] -> w581
          tunnel: w580 -> [w588 w595 w607]
          tunnel: [w587 w594 w608] -> w579
          tunnel: w578 -> [w585 w591 w605]
          tunnel: [w584 w590 w604] -> w577
          event Timeout {
            n144 = event-data() -> ()  [unwired: 1 in, 3 out]
            n145 = Enqueue Element(queue=w588, element=TLB_event_states."Idle" ("Enum"), error in (no error)=w585) -> (queue out=w587:refnum<queue>, error out=w584:errorcluster)  [unwired: 1 in, 1 out]
          }
          event User Event {
            n146 = event-data() -> ()  [unwired: 1 in, 5 out]
            n147 = case shown="Default" "Tasks Selector" {
              tunnel: [TLB_event_states."Idle" ("Enum") TLB_event_states."Start Task 1" ("Enum") TLB_event_states."Start Task 2" ("Enum") TLB_event_states."Start Task 3" ("Enum") TLB_event_states."Start Task 4" ("Enum") TLB_event_states."Wall follow mode" ("Enum") TLB_event_states."Camera vision" ("Enum")] -> w592
              frame Default {
              }
              frame "Task 1" {
              }
              frame "Task 2" {
              }
              frame "Task 3" {
              }
              frame "Task 4" {
              }
              frame "Wall following" {
              }
              frame "RT Camera tracking" {
              }
            }
            n148 = Enqueue Element(queue=w595, element=w592, error in (no error)=w591) -> (queue out=w594:refnum<queue>, error out=w590:errorcluster)  [unwired: 1 in, 1 out]
          }
          event User Event {
            n149 = event-data() -> ("Stop Queue"=w609:bool)  [unwired: 1 in, 4 out]
            n150 = Enqueue Element At Opposite End(queue=w607, element=TLB_event_states."Exit" ("Enum"), error in (no error)=w605) -> (queue out=w608:refnum<queue>, error out=w604:errorcluster)  [unwired: 1 in, 1 out]
          }
        }
        "Event handling loop" <- w576
      }
      n151 = while {
        tunnel: w37 -> [w622]
        tunnel: w38 -> [w621]
        tunnel: [w620] -> w44
        tunnel: [w619] -> w43
        tunnel: w42 -> [w618]
        tunnel: [w617] -> w40
        tunnel: w41 -> [w616]
        tunnel: [w615] -> w39
        i -> [w612]
        stop <- w613 stop-if-true
        # "Generate USER Event Loop"
        n152 = local read "DIO 0"() -> (w611:bool)
        n153 = case shown="True" w611 {
          selector: w611 -> [_ w634]
          tunnel: w622 -> [w633 w638]
          tunnel: [w633 w637] -> w619
          tunnel: w618 -> [w632 w636]
          tunnel: [w632 w635] -> w617
          frame False {
          }
          frame True {
            n154 = Generate User Event(user event=w638, event data cluster=w634, error in=w636) -> (user event out=w637:refnum<user-event>, error out=w635:errorcluster)  [unwired: 1 in]
          }
        }
        n155 = case shown="False" "STOP" {
          selector: "STOP" -> [_ w627]
          tunnel: w621 -> [w626 w631]
          tunnel: [w626 w630] -> w620
          tunnel: w616 -> [w625 w629]
          tunnel: [w625 w628] -> w615
          tunnel: [FALSE w627] -> w613
          frame False {
          }
          frame True {
            n156 = Generate User Event(user event=w631, event data cluster=w627, error in=w629) -> (user event out=w630:refnum<user-event>, error out=w628:errorcluster)  [unwired: 1 in]
          }
        }
        n157 = call "FGV Stop.vi"("Init/Read/Write State"=States_for_Action_Engine."Write", "Input Node"=w613) -> ()  [unwired: 1 in, 2 out]
        n158 = Wait (ms)(milliseconds to wait=u32 20) -> ()  [unwired: 1 out]
        "User event loop" <- w612
      }
      n159 = while {
        i -> [w98]
        stop <- w110 stop-if-true
        w100 = 50 ("sample length")
        w115 = T22 [enum."A/AI0"] items=["Not Connected", "AudioIn/Left", "AudioIn/Right", "C/AI0", "C/AI1", "A/AI0", "A/AI1", "A/AI2", "A/AI3", "A/AI4", "A/AI5", "A/AI6", "A/AI7", "B/AI0", "B/AI1", "B/AI2", "B/AI3", "B/AI4", "B/AI5", "B/AI6", "B/AI7", "AI/AI0", "AI/AI1", "AI/AI2", "AI/AI3", "A/AI0 (DIFF)", "A/AI1 (DIFF)", "A/AI2 (DIFF)", "A/AI3 (DIFF)", "B/AI0 (DIFF)", "B/AI1 (DIFF)", "B/AI2 (DIFF)", "B/AI3 (DIFF)"] ("AI Channel")
        w116 = T22 [enum."B/AI0"] items=["Not Connected", "AudioIn/Left", "AudioIn/Right", "C/AI0", "C/AI1", "A/AI0", "A/AI1", "A/AI2", "A/AI3", "A/AI4", "A/AI5", "A/AI6", "A/AI7", "B/AI0", "B/AI1", "B/AI2", "B/AI3", "B/AI4", "B/AI5", "B/AI6", "B/AI7", "AI/AI0", "AI/AI1", "AI/AI2", "AI/AI3", "A/AI0 (DIFF)", "A/AI1 (DIFF)", "A/AI2 (DIFF)", "A/AI3 (DIFF)", "B/AI0 (DIFF)", "B/AI1 (DIFF)", "B/AI2 (DIFF)", "B/AI3 (DIFF)"] ("AI Channel")
        # "IR + Ultrasonic Sensor Loop"
        n160 = call <vilib>:"Ping.vi"("Mxp Side"=Mxp_Selection."MXP B") -> ("CM"=w104:fxp<+,64,16>)  [unwired: 8 in, 2 out]
        "Right Ultrasonic" <- w104
        n161 = call <vilib>:"Ping.vi"("Mxp Side"=Mxp_Selection."MXP A") -> ("CM"=w105:fxp<+,64,16>)  [unwired: 8 in, 2 out]
        "Left Ultrasonic" <- w105
        n162 = call <vilib>:"Sharp IR.vi"("AI Channel"=w116) -> ("Sharp IR Distance"=→"Right IR Sensor":dbl)  [unwired: 8 in, 2 out]
        n163 = call <vilib>:"Sharp IR.vi"("AI Channel"=w115) -> ("Sharp IR Distance"=→"Left IR Sensor":dbl)  [unwired: 8 in, 2 out]
        n164 = Add(x=w105, y=w104) -> (x+y=w107:fxp<+,64,17>)
        n165 = Divide(x=w107, y=fxp<+,64,17> 2.0) -> (x/y=w103:fxp<+,64,64>)
        n166 = call "FGV Stop.vi"("Init/Read/Write State"=States_for_Action_Engine."Read") -> ("Output node"=w110:bool)  [unwired: 2 in, 1 out]
        n167 = call <vilib>:"Median PtByPt.vi"("sample length"=w100, "x"=w103) -> ("median"=w102:dbl)  [unwired: 2 in, 1 out]
        n168 = call <vilib>:"Mode PtByPt.vi"("sample length"=w100, "intervals"=50, "x"=w102) -> ("mode"=→"L/R average":dbl)  [unwired: 1 in, 1 out]
        n169 = Wait Until Next ms Multiple(millisecond multiple=u32 20) -> ()  [unwired: 1 out]
        "Sensor Loop" <- w98
      }
      n170 = while {
        tunnel: [w90] -> w18
        i -> [w82]
        stop <- w92 stop-if-true
        # "NavX Loop"
        n171 = call <vilib>:"NavX Open.vi"("I2C Channel"=I2C_Channel."A") -> ("NavX Info"=w83:T7)  [unwired: 9 in, 1 out]
        n172 = case shown="True" "NavX Zero Yaw" {
          tunnel: w83 -> [w94 w96]
          tunnel: [w94 w95] -> _
          frame False {
          }
          frame True {
            n173 = call <vilib>:"Zero Yaw.vi"("NavX Info In"=w96) -> ("NavX Info Out"=w95:T7)  [unwired: 10 in]
          }
        }
        n174 = call <vilib>:"YRPHfH.vi"("NavX Info In"=w83) -> ("YRPHfH"=w86:T10)  [unwired: 3 in, 1 out]
        "YRPHfH" <- w86
        n175 = call <vilib>:"Raw Values.vi"("NavX Info In"=w83) -> ("NavX Info Out"=w90:T7)  [unwired: 8 in, 1 out]
        "NavX Info Out" <- w90
        n176 = call <vilib>:"LinearAcceleration.vi"("NavX Info In"=w83) -> ("LinearAcceleration"=→"LinearAcceleration":T8)  [unwired: 9 in, 1 out]
        n177 = call <vilib>:"Displacement.vi"("NavX Info In"=w83) -> ("Displacement"=→"Displacement":T9)  [unwired: 9 in, 1 out]
        n178 = Unbundle By Name(w86) -> ("Yaw"=→"Yaw":dbl)
        n179 = call "FGV Stop.vi"("Init/Read/Write State"=States_for_Action_Engine."Read") -> ("Output node"=w92:bool)  [unwired: 2 in, 1 out]
        n180 = Wait Until Next ms Multiple(millisecond multiple=u32 10) -> ()  [unwired: 1 out]
        "NavX Loop" <- w82
      }
      n181 = while {
        tunnel: w16 -> [w61]
        tunnel: [w60] -> w15
        tunnel: w12 -> [w59]
        tunnel: [w58] -> w11
        tunnel: w10 -> [w57]
        tunnel: [w56] -> w9
        tunnel: w8 -> [w55]
        tunnel: [w54] -> w7
        i -> [w66]
        stop <- w76 stop-if-true
        # "Blackhawk interfacing"
        n182 = call <vilib>:"Blackhawk i2c Open.vi"("I2C Channel"=I2C_Channel."B") -> ("I2C Ref Out"=w81:T24, "error out"=w80:errorcluster)  [unwired: 2 in]
        n183 = call <vilib>:"Blackhawk DIO Read.vi"("I2C Ref In"=w81, "PIN"=u8 0, "error in (no error)"=w80) -> ("I2C Ref Out"=w74:T24, "error out"=w75:errorcluster)  [unwired: 3 in, 1 out]
        n184 = call <vilib>:"C DIO Read.vi"("error in (no error)"=w55, "DIO Info In in"=w59) -> ("error out"=w54:errorcluster, "IN"=→"DIO 1":bool, "DIO Info In out"=w58:T20)  [unwired: 7 in]
        n185 = call <vilib>:"C DIO Read.vi"("error in (no error)"=w57, "DIO Info In in"=w61) -> ("error out"=w56:errorcluster, "IN"=→"DIO 0":bool, "DIO Info In out"=w60:T20)  [unwired: 7 in]
        n186 = call <vilib>:"Blackhawk Relay.vi"("error in (no error)"=w75, "On/Off"="On/Off", "Relay"=enum8{"Relay 0", "Relay 1", "Relay 2"}."Relay 0", "I2C Ref In"=w74) -> ("error out"=w71:errorcluster, "I2C Ref Out"=w68:T24)  [unwired: 6 in]
        n187 = call <vilib>:"Blackhawk Servo.vi"("error in (no error)"=w71, "Servo Select"=enum16{"Servo 5", "Servo 6"}."Servo 5", "Servo Angle"="Servo Angle", "I2C Ref In"=w68) -> ("error out"=w65:errorcluster, "I2C Ref Out"=w64:T24)  [unwired: 6 in]
        n188 = call <vilib>:"Blackhawk read Limit.vi"("error in (no error)"=w65, "I2C Ref In"=w64) -> ("error out"=→"Blackhawk error":errorcluster, "Limit Switch Array"=→"Limit Switch Array":bool[])  [unwired: 1 in, 1 out]
        n189 = call "FGV Stop.vi"("Init/Read/Write State"=States_for_Action_Engine."Read") -> ("Output node"=w76:bool)  [unwired: 2 in, 1 out]
        n190 = Wait (ms)(milliseconds to wait=u32 20) -> ()  [unwired: 1 out]
        "Blackhawk loop" <- w66
      }
      n191 = while {
        tunnel: w23 -> [w126]
        tunnel: w22 -> [w123]
        i -> [w117]
        stop <- w120 stop-if-true
        # "Status Loop for Action Queues"
        n192 = Get Queue Status(queue=w126, return elements? (F)=TRUE) -> (error out=w122:errorcluster, # elements in queue=→"Action Queue Items":i32, elements=→"Action Queues items":string[])  [unwired: 1 in, 5 out]
        n193 = Get Queue Status(queue=w123, return elements? (F)=TRUE) -> (# pending remove=→"State Logic Queue Items":i32, error out=w121:errorcluster)  [unwired: 1 in, 6 out]
        n194 = Merge Errors(w122, w121) -> (w120:errorcluster)
        n195 = Wait (ms)(milliseconds to wait=u32 500) -> ()  [unwired: 1 out]
        "Status loop" <- w117
      }
      n196 = call <vilib>:"DIO Close.vi"("error in (no error)"=w9, "DIO Info In"=w15) -> ()  [unwired: 9 in, 1 out]
      n197 = call <vilib>:"DIO Close.vi"("error in (no error)"=w7, "DIO Info In"=w11) -> ()  [unwired: 9 in, 1 out]
      n198 = while {
        stop <- w49 stop-if-true
        # "Motor Control Loop"
        n199 = Wait Until Next ms Multiple(millisecond multiple=u32 5) -> ()  [unwired: 1 out]
        n200 = call "New motor Control integrated remodeled.vi"("States"=enum16{"RESET ENCODER", "WRITE", "READ", "INIT"}."READ") -> ("Speed and distance cluster"=→"Speed and distance cluster":T1)  [unwired: 4 in, 1 out]
        n201 = call "FGV Stop.vi"("Init/Read/Write State"=States_for_Action_Engine."Read") -> ("Output node"=w49:bool)  [unwired: 2 in, 1 out]
      }
      n202 = call <vilib>:"NavX Close.vi"("NavX Info In"=w18) -> ()  [unwired: 10 in, 1 out]
      n203 = Merge Errors "Merge Errors"(w40, w39) -> (w21:errorcluster)
      n204 = Merge Errors(w25, w21) -> (w4:errorcluster)
      n205 = Destroy User Event(user event=w43, error in=w4) -> ()  [unwired: 1 out]
      n206 = Destroy User Event(user event=w44, error in=w4) -> ()  [unwired: 1 out]
      n207 = Unregister For Events(event registration refnum=w35, error in=w4) -> ()  [unwired: 1 out]
      n208 = Release Queue(queue=w6, error in (no error)=w4) -> (error out=→"error out":errorcluster)  [unwired: 1 in, 2 out]
      n209 = Release Queue(queue=w34, error in (no error)=w4) -> ()  [unwired: 1 in, 3 out]
    }
    frame #2 {
      n210 = call "New motor Control integrated remodeled.vi"("States"=enum16{"RESET ENCODER", "WRITE", "READ", "INIT"}."WRITE", "Target Speed"=T19 {"xTargetSpeed"=0.0, "yTargetSpeed"=0.0, "wTargetSpeed"=0.0}) -> ()  [unwired: 3 in, 2 out]
    }
    frame #3 {
    }
  }
